vi "打开数据文件夹.vi"   [LabVIEW 2020]
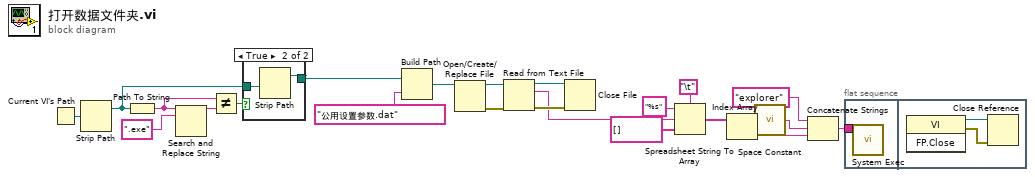
[diagram p0: block diagram]
diagram:
  n1 = Current VI's Path() -> (path=w15:path)
  n2 = Strip Path(path=w15) -> (stripped path=w10:path)  [unwired: 1 out]
  n3 = Path To String(path=w10) -> (string=w12:string)
  n4 = Search and Replace String(input string=w12, search string=".exe" ("搜索字符串")) -> (result string=w13:string)  [unwired: 6 in, 3 out]
  n5 = Not Equal?(x=w12, y=w13) -> (x != y?=w11:bool)
  n6 = case shown="True" w11 {
    tunnel: w10 -> [w23 w24]
    tunnel: [w23 w25] -> w9
    frame False {
    }
    frame True {
      n7 = Strip Path(path=w24) -> (stripped path=w25:path)  [unwired: 1 out]
    }
  }
  n8 = Build Path(base path=w9, name or relative path="公用设置参数.dat") -> (appended path=w18:path)
  n9 = Open/Create/Replace File(file path (use dialog)=w18) -> (refnum out=w8:refnum<file>, error out=w7:errorcluster)  [unwired: 5 in, 1 out]
  n10 = Read from Text File(file (use dialog)=w8, error in=w7) -> (refnum out=w16:refnum<file>, text=w3:string, error out=w17:errorcluster)  [unwired: 1 in, 2 out]
  n11 = Close File(refnum=w16, error in=w17) -> ()  [unwired: 2 out]
  n12 = Spreadsheet String To Array(delimiter (Tab)="\t", format string="%s", spreadsheet string=w3, array type (2D Dbl)=string[] [] ("添加的数组")) -> (array=w2:string[])
  n13 = Index Array(array=w2) -> (element=w1:string)  [unwired: 1 in]
  n14 = call <vilib>:"Space Constant.vi"() -> ("String"=w22:string)
  n15 = Concatenate Strings("explorer" ("字符串"), w22, w1) -> (w20:string)
  n16 = flat-sequence {
    tunnel: w20 -> [w26]
    frame #0 {
      n17 = call <vilib>:"System Exec.vi"("command line"=w26) -> ()  [unwired: 7 in, 4 out]
    }
    frame #1 {
      n18 = invoke class="VI" method="FP.Close"() -> (reference out=w27:refnum<vi>, error out=w28:errorcluster)  [unwired: 3 in, 1 out]
      n19 = Close Reference(reference=w27, error in (no error)=w28) -> ()  [unwired: 1 out]
    }
  }
